vi "server-全局变量.vi"() -> ()   [LabVIEW 2013]
panel:
  out "服务器引用层次":T1
  out "侦听Port":u16=60000
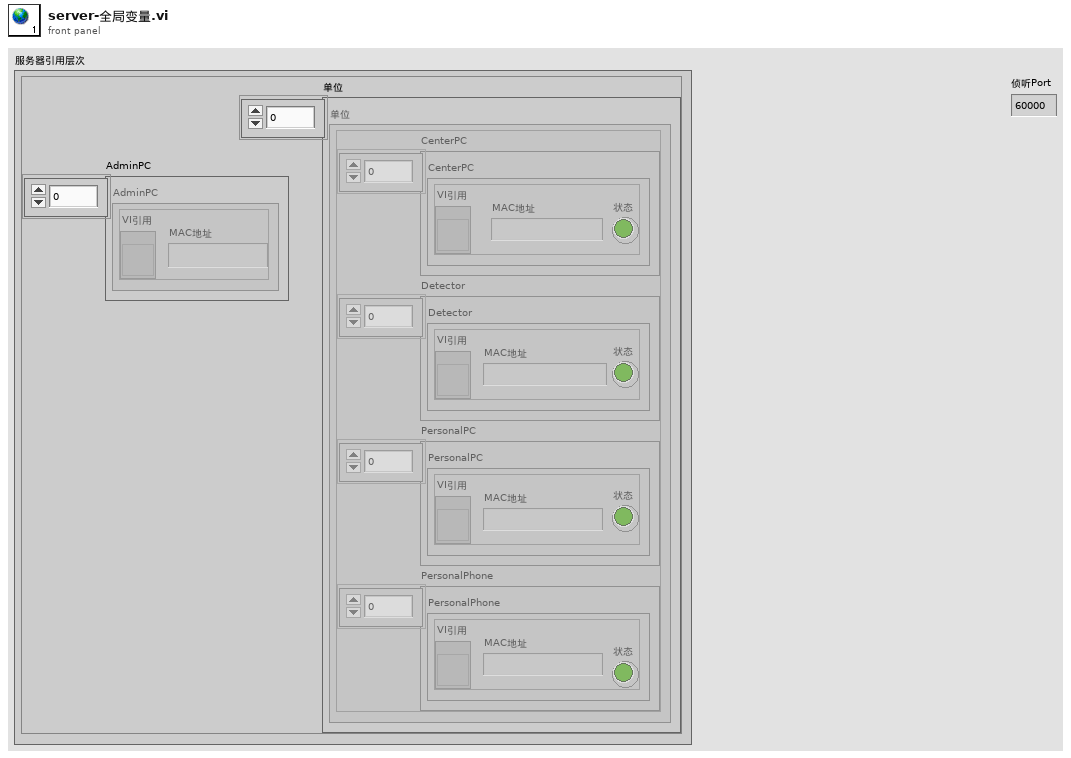
[diagram p1: front panel]
types:
  T1 = cluster{"单位":cluster{"CenterPC":cluster{"VI引用":refnum<vi>, "MAC地址":string, "状态":bool}[], "Detector":cluster{"VI引用":refnum<vi>, "MAC地址":string, "状态":bool}[], "PersonalPC":cluster{"VI引用":refnum<vi>, "MAC地址":string, "状态":bool}[], "PersonalPhone":cluster{"VI引用":refnum<vi>, "MAC地址":string, "状态":bool}[]}[], "AdminPC":cluster{"VI引用":refnum<vi>, "MAC地址":string}[]}
diagram:
